vi "Init Front Panel Ctrls.vi"(8 "error in":errorcluster, 10 "Latest Loop Count":i32, 11 "Ctrl Ref":T1) -> (0 "error out":errorcluster)   [LabVIEW 2020, in "GUCalibration2.lvlib"]
uses:
  GUCalibration2.lvlib
  Controls/GU Arrange UI Ref.ctl
  <vilib>/Utility/miscctls.llb/LVBoundsTypeDef.ctl
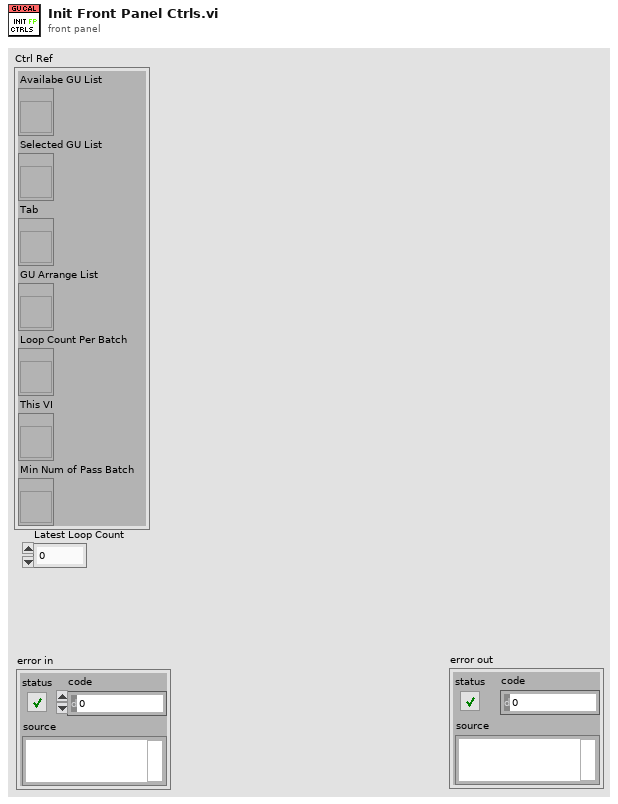
[diagram p1: front panel]
types:
  T1 = typedef "GUCalibration2.lvlib/GU Arrange UI Ref.ctl" = cluster{"Availabe GU List":refnum<vi>, "Selected GU List":refnum<vi>, "Tab":refnum<vi>, "GU Arrange List":refnum<vi>, "Loop Count Per Batch":refnum<vi>, "This VI":refnum<vi>, "Min Num of Pass Batch":refnum<vi>}
  T2 = typedef "LVBoundsTypeDef.ctl" = cluster{"Width":u32, "Height":u32}
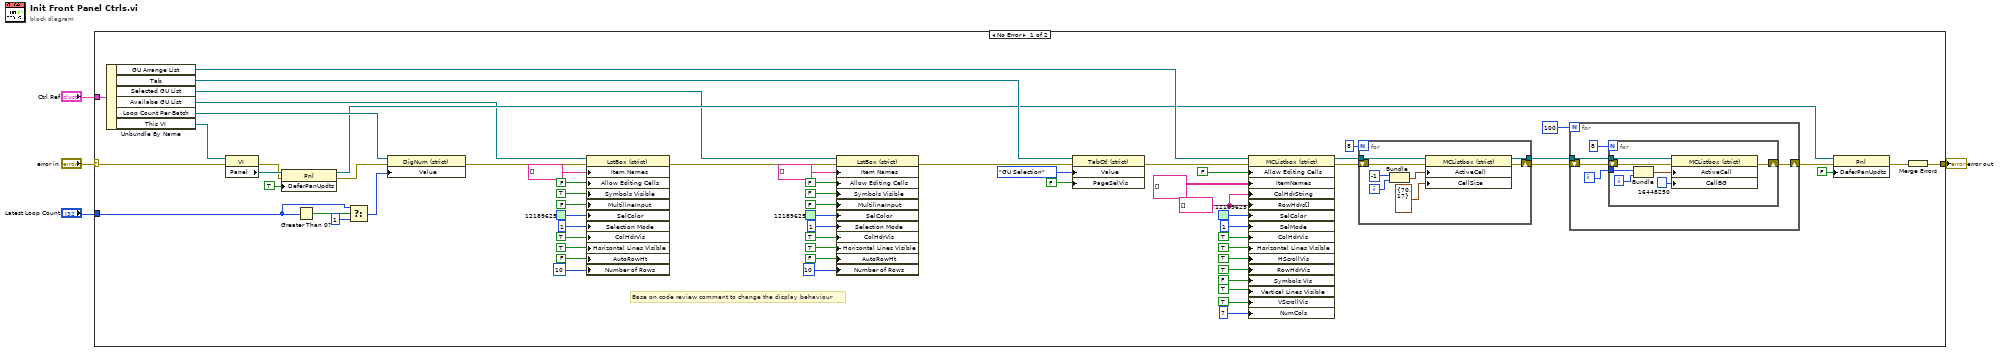
[diagram p0: block diagram]
diagram:
  n1 = case shown="No Error" "error in" {
    selector: "error in" -> [w47 w91]
    tunnel: "Ctrl Ref" -> [w70 _]
    tunnel: [w69 w91] -> w3
    tunnel: "Latest Loop Count" -> [w29 _]
    frame No Error {
      w61 = string[] [] ("Column Header Strings[]")
      # "Base on code review comment to change the display behaviour"
      n2 = Unbundle By Name(w70) -> ("GU Arrange List"=w65:refnum<vi>, "Tab"=w68:refnum<vi>, "Selected GU List"=w27:refnum<vi>, "Availabe GU List"=w6:refnum<vi>, "Loop Count Per Batch"=w51:refnum<vi>, "This VI"=w48:refnum<vi>)
      n3 = property class="VI"(reference=w48, error in=w47) -> (error out=w43:errorcluster, "Panel"=w46:refnum<vi>)  [unwired: 1 out]
      n4 = property class="Pnl"(reference=w46, error in=w43, "DeferPanUpdts"=TRUE ("Defer Panel Updates")) -> (reference out=w39:refnum<vi>, error out=w44:errorcluster)
      n5 = Greater Than 0?(x=w29) -> (x > 0?=w32:bool)
      n6 = Select(t=w29, s=w32, f=1) -> (s? t:f=w30:i32)
      n7 = property class="DigNum (strict)"(reference=w51, error in=w44, "Value"=w30) -> (error out=w50:errorcluster)  [unwired: 1 out]
      n8 = property class="LstBox (strict)"(reference=w6, error in=w50, "Item Names"=string[] [], "Allow Editing Cells"=FALSE, "Symbols Visible"=TRUE ("Visible Items:Symbols Visible"), "MultilineInput"=FALSE ("Multiple Line Input"), "SelColor"=u32 12189625, "Selection Mode"=1, "ColHdrVis"=TRUE ("Visible Items:Column Header Visible"), "Horizontal Lines Visible"=TRUE ("Visible Items:Horizontal Lines Visible"), "AutoRowHt"=FALSE ("Autosizing Row Height"), "Number of Rows"=u32 10) -> (error out=w28:errorcluster)  [unwired: 1 out]
      n9 = property class="LstBox (strict)"(reference=w27, error in=w28, "Item Names"=string[] [], "Allow Editing Cells"=FALSE, "Symbols Visible"=FALSE ("Visible Items:Symbols Visible"), "MultilineInput"=FALSE ("Multiple Line Input"), "SelColor"=u32 12189625, "Selection Mode"=1, "ColHdrVis"=TRUE ("Visible Items:Column Header Visible"), "Horizontal Lines Visible"=TRUE ("Visible Items:Horizontal Lines Visible"), "AutoRowHt"=FALSE ("Autosizing Row Height"), "Number of Rows"=u32 10) -> (error out=w5:errorcluster)  [unwired: 1 out]
      n10 = property class="TabCtl (strict)"(reference=w68, error in=w5, "Value"=enum32{"GU Selection", "GU Distribution"}."GU Selection", "PageSelVis"=FALSE ("Page Selector Visible")) -> (error out=w64:errorcluster)  [unwired: 1 out]
      n11 = property class="MCListbox (strict)"(reference=w65, error in=w64, "Allow Editing Cells"=FALSE, "ItemNames"=string[][] [] ("Item Names"), "ColHdrString"=w61, "RowHdrs[]"=w61, "SelColor"=u32 12189625, "SelMode"=1 ("Selection Mode"), "ColHdrVis"=TRUE ("Visible Items:Column Headers Visible"), "Horizontal Lines Visible"=TRUE ("Visible Items:Horizontal Lines Visible"), "HScrollVis"=TRUE ("Visible Items:Horizontal Scrollbar Visible"), "RowHdrVis"=TRUE ("Visible Items:Row Headers Visible"), "Symbols Vis"=FALSE ("Visible Items:Symbols Visible"), "Vertical Lines Visible"=TRUE ("Visible Items:Vertical Lines Visible"), "VScrollVis"=TRUE ("Visible Items:Vertical Scrollbar Visible"), "NumCols"=u32 7 ("Number of Rows")) -> (reference out=w38:refnum<vi>, error out=w37:errorcluster)
      n12 = for {
        N: 8 -> [_]
        shift-right: [w74] -> w36
        shift-left: w37 -> [w77]
        tunnel: w38 -> [w78]
        tunnel: [w71] -> w35
        i -> [w76]
        n13 = Bundle("Row"=-1, w76) -> (w75:cluster{"Row":i32, i32})  [unwired: 1 in]
        n14 = property class="MCListbox (strict)"(reference=w78, error in=w77, "ActiveCell"=w75, "CellSize"=T2 {"Width"=70, "Height"=17} ("Active Cell:Cell Size 2")) -> (reference out=w71:refnum<vi>, error out=w74:errorcluster)
      }
      n15 = for {
        N: 100 -> [_]
        tunnel: w35 -> [w83]
        shift-right: [w79] -> w41
        shift-left: w36 -> [w82]
        i -> [w81]
        n16 = for {
          N: 8 -> [_]
          tunnel: w83 -> [w90]
          tunnel: w81 -> [w88]
          shift-right: [w84] -> w79
          shift-left: w82 -> [w89]
          i -> [w87]
          n17 = Bundle(w88, w87) -> (w86:cluster{i32, i32})  [unwired: 1 in]
          n18 = property class="MCListbox (strict)"(reference=w90, error in=w89, "ActiveCell"=w86, "CellBG"=u32 16448250) -> (error out=w84:errorcluster)  [unwired: 1 out]
        }
      }
      n19 = property class="Pnl"(reference=w39, error in=w41, "DeferPanUpdts"=FALSE ("Defer Panel Updates")) -> (error out=w40:errorcluster)  [unwired: 1 out]
      n20 = Merge Errors(w40) -> (w69:errorcluster)
    }
    frame Error {
    }
  }
  "error out" <- w3
